vi "Scanner.vi"(9 "Continuous":bool, 10 "IntGraph Refnum":refnum<vi>, 11 "Scan Parameters":T1 {"Dwell Time (ms)" min=0; "Y Step" min=0.0; "X Step" min=0.0}) -> (3 "Counts":i32[][](array[numeric]))   [LabVIEW 2012]
uses:
  Strict Type Def - Scan Parameters Cluster.ctl
  <vilib>/DAQmx/write.llb/DAQmx Write (Analog DBL 1Chan 1Samp).vi
  Channels.vi
  <vilib>/DAQmx/create/channels.llb/DAQmx Create Channel (AO-Voltage-Basic).vi
  Global Vars.vi
  <vilib>/DAQmx/miscellaneous.llb/DAQmx Fill In Error Info.vi
panel:
  out "A0 Voltage":dbl caption="A1 Voltage"
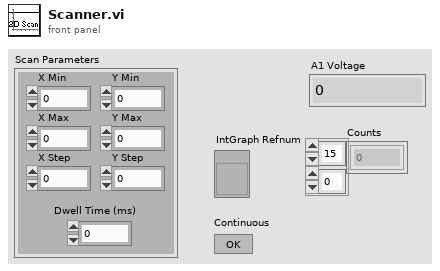
[diagram p1: front panel]
types:
  T1 = typedef "Strict Type Def - Scan Parameters Cluster.ctl" = cluster{"X Max":dbl, "X Min":dbl, "X Step":dbl, "Y Max":dbl, "Y Min":dbl, "Y Step":dbl, "Dwell Time (ms) ":i32}
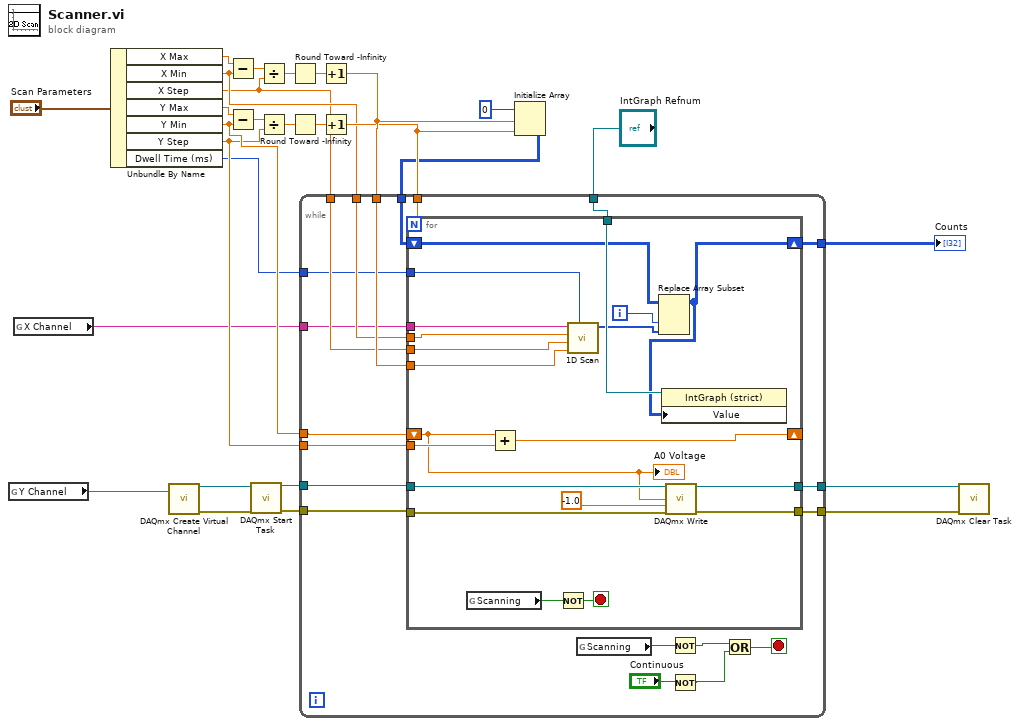
[diagram p0: block diagram]
diagram:
  n1 = global read "Channels.vi" "Y Channel"() -> (w6:tag)
  n2 = global read "Channels.vi" "X Channel"() -> (w5:tag)
  n3 = Unbundle By Name("Scan Parameters") -> ("X Max"=w16:dbl, "X Min"=w15:dbl, "X Step"=w14:dbl, "Y Max"=w13:dbl, "Y Min"=w12:dbl, "Y Step"=w11:dbl, "Dwell Time (ms)"=w10:i32)
  n4 = call-poly <vilib>:"DAQmx Create Virtual Channel.vi"("physical channels"=w6) -> ("task out"=w4:refnum<k21>, "error out"=w3:errorcluster)  [unwired: 13 in]
  n5 = Subtract(x=w16, y=w15) -> (x-y=w28:dbl)
  n6 = Subtract(x=w13, y=w12) -> (x-y=w27:dbl)
  n7 = call <vilib>:"DAQmx Start Task.vi"("task/channels in"=w4, "error in"=w3) -> ("task out"=w2:refnum<k21>, "error out"=w1:errorcluster)  [unwired: 12 in]
  n8 = Divide(x=w28, y=w14) -> (x/y=w24:dbl)
  n9 = Divide(x=w27, y=w11) -> (x/y=w23:dbl)
  n10 = Round Toward -Infinity(1:w24) -> (0:w21:dbl)
  n11 = Round Toward -Infinity(1:w23) -> (0:w20:dbl)
  n12 = Increment(x=w21) -> (x+1=w19:dbl)
  n13 = Increment(x=w20) -> (x+1=w18:dbl)
  n14 = Initialize Array(u32 0 ("element"), w19, w18) -> (w8:u32[][])
  n15 = while {
    tunnel: [w48] -> w26
    tunnel: [w47] -> w25
    tunnel: w19 -> [w46]
    tunnel: w18 -> [w45]
    tunnel: w15 -> [w44]
    tunnel: w14 -> [w43]
    tunnel: w12 -> [w42]
    tunnel: w11 -> [w41]
    tunnel: w10 -> [w40]
    tunnel: "IntGraph Refnum" -> [w39]
    tunnel: w8 -> [w38]
    tunnel: [w37] -> w7
    tunnel: w5 -> [w36]
    tunnel: w2 -> [w35]
    tunnel: w1 -> [w34]
    stop <- w33 stop-if-true
    n16 = for {
      N: w45 -> [_]
      shift-right: [w68] -> _
      shift-left: w42 -> [w61]
      tunnel: [w66] -> w48
      tunnel: [w65] -> w47
      tunnel: w35 -> [w64]
      tunnel: w34 -> [w63]
      tunnel: w44 -> [w57]
      tunnel: w43 -> [w56]
      tunnel: w41 -> [w62]
      tunnel: w46 -> [w55]
      tunnel: w40 -> [w59]
      tunnel: w39 -> [w60]
      tunnel: w36 -> [w58]
      shift-right: [w52] -> w37
      shift-left: w38 -> [w54]
      i -> [w51]
      stop <- w49 stop-if-true
      n17 = global read "Global Vars.vi" "Scanning"() -> (w50:bool)
      n18 = Add(x=w61, y=w62) -> (x+y=w68:dbl)
      n19 = Not(x=w50) -> (.not. x?=w49:bool)
      n20 = call "1D Scan.vi"("Dwell Time (ms)"=w59, "Num Steps"=w55, "Step"=w56, "Min"=w57, "Channel"=w58) -> ("Counts"=w53:i32[])  [unwired: 6 in]
      n21 = Replace Array Subset(array=w54, new element=w53, index (col)=w51) -> (w52:u32[][])  [unwired: 1 in]
      n22 = property class="IntGraph (strict)"(reference=w60, "Value"=w52) -> ()  [unwired: 1 in, 2 out]
      n23 = call-poly <vilib>:"DAQmx Write.vi"("task/channels in"=w64, "data"=w61, "timeout"=-1.0, "error in"=w63) -> ("task out"=w66:refnum<k21>, "error out"=w65:errorcluster)  [unwired: 9 in, 1 out]
      "A0 Voltage" <- w61
    }
    n24 = global read "Global Vars.vi" "Scanning"() -> (w32:bool)
    n25 = Not(x=w32) -> (.not. x?=w31:bool)
    n26 = Not(x="Continuous") -> (.not. x?=w29:bool)
    n27 = Or(x=w31, y=w29) -> (x .or. y?=w33:bool)
  }
  "Counts" <- w7
  n28 = call <vilib>:"DAQmx Clear Task.vi"("task in"=w26, "error in"=w25) -> ()  [unwired: 13 in, 1 out]
